vi "Oscillation_of_MCL_Host-AidanHamilton.vi"() -> ()   [LabVIEW 2012]
uses:
  <vilib>/FPGAPlugInAG/PCI-7831R/niLvFpga_Open_PCI-7831R.vi
  <vilib>/rvi/interface/common/dynamic/niFpgaDynamicAddResources.vi
  <vilib>/Utility/error.llb/Error Cluster From Error Code.vi
  <vilib>/rvi/errors/niLvFpgaAdjustHostInterfaceError.vi
  <vilib>/FPGAPlugInAG/Dynamic/niLvFpga_Close_Dynamic.vi
  <vilib>/rvi/interface/nirviOpenFPGA/nirviOpenFPGA.xnode
  SB130-XPS/Documents/FPGA-project-apporach-retraction/FPGA Bitfiles/Apporach-Retract_FPGATarget2_OscillationofMCL_BWtLzaB8-Ng.lvbitx
  Oscillation_of_MCL_Target-AidanHamiltontestcopy.vi
  <vilib>/rvi/interface/nirviReadWriteControl/nirviReadWriteControl.xnode
  <vilib>/rvi/interface/nirviCloseFPGA/nirviCloseFPGA.xnode
  NiFpgaLv.dll
  <vilib>/rvi/interface/Simulation/niFpgaSimulationCallBeginRW.vi
panel:
  out "Numeric":i16
  in  "Oscillation (on/off)":bool
  in  "Frequency (Hz)":i32
  in  "Amplitude  (nm)":i16
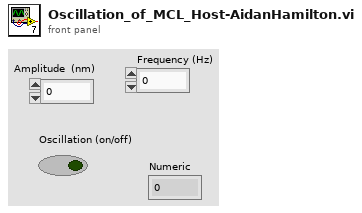
[diagram p1: front panel]
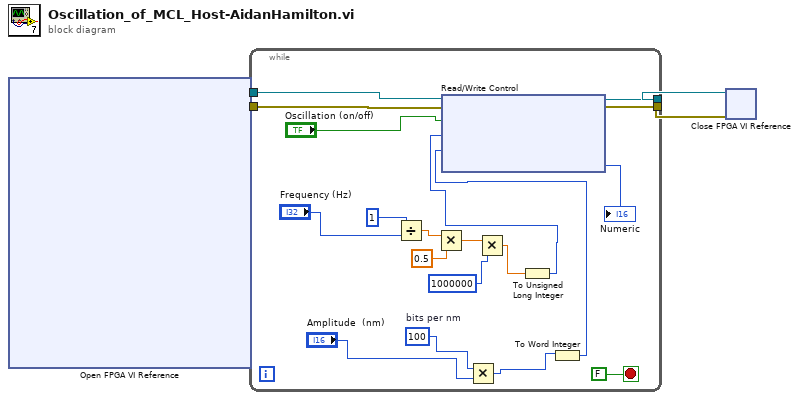
[diagram p0: block diagram]
diagram:
  n1 = xnode "Open FPGA VI Reference"() -> ("FPGA VI Reference Out"=w4:refnum<k20>, "error out"=w1:errorcluster)  [unwired: 2 in]
  n2 = while {
    tunnel: w4 -> [w11]
    tunnel: [w23] -> w3
    tunnel: w1 -> [w15]
    tunnel: [w14] -> w2
    stop <- FALSE stop-if-true
    w5 = 100  # bits per nm
    n3 = Divide(x=1, y="Frequency (Hz)") -> (x/y=w20:dbl)
    n4 = Multiply(x=w20, y=0.5) -> (x*y=w17:dbl)
    n5 = Multiply(x=w5, y="Amplitude  (nm)") -> (x*y=w12:i32)
    n6 = Multiply(x=w17, y=1000000) -> (x*y=w8:dbl)
    n7 = To Unsigned Long Integer(number=w8) -> (unsigned 32bit integer=w7:u32)
    n8 = To Word Integer(number=w12) -> (16bit integer=w9:i16)
    n9 = xnode "Read/Write Control"("FPGA VI Reference In"=w11, "error in"=w15, "Oscillation on/off"="Oscillation (on/off)", "1/2 the period of oscillation"=w7, "Amplitude"=w9) -> ("FPGA VI Reference Out"=w23:refnum<k20>, "error out"=w14:errorcluster, "Numeric"=→"Numeric":u64)
  }
  n10 = xnode "Close FPGA VI Reference"("FPGA VI Reference In"=w3, "error in"=w2) -> ()  [unwired: 1 out]
